vi "Agilent34410A Get Apperture.vi"(8 "error in (no error)":errorcluster, 10 "DMM Function":T2, 11 "VISA Rsrc":refnum<visa-resource-name>="SR530") -> (0 "error out":errorcluster, 1 "Aperture (s)":dbl, 2 "NPLC Val":dbl, 3 "VISA Rsrc Out":refnum<visa-resource-name>="GPIB0::12::INSTR", 4 "ChaineRep":string caption="Chaîne de Réponse", 5 "Apperture Enable":bool caption="App Enable", 6 "NPLC":T1(ring))   [LabVIEW 2019]
uses:
  <userlib>/Agilent34410A/Agilent34410A DMM_Func.ctl
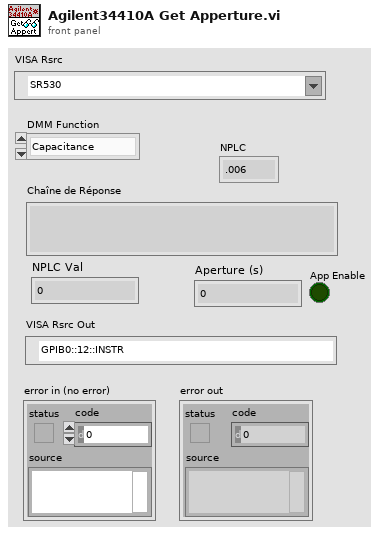
[diagram p1: front panel]
types:
  T1 = enum16{".006", ".02", ".06", ".2", "1", "2", "10", "100"}
  T2 = typedef "Agilent34410A DMM_Func.ctl" = enum16{"Capacitance", "Continuity", "Current AC", "Current", "Diode", "Frequency", "4W Resistance", "Period", "Resistance", "Temperature", "Voltage AC", "Voltage"}
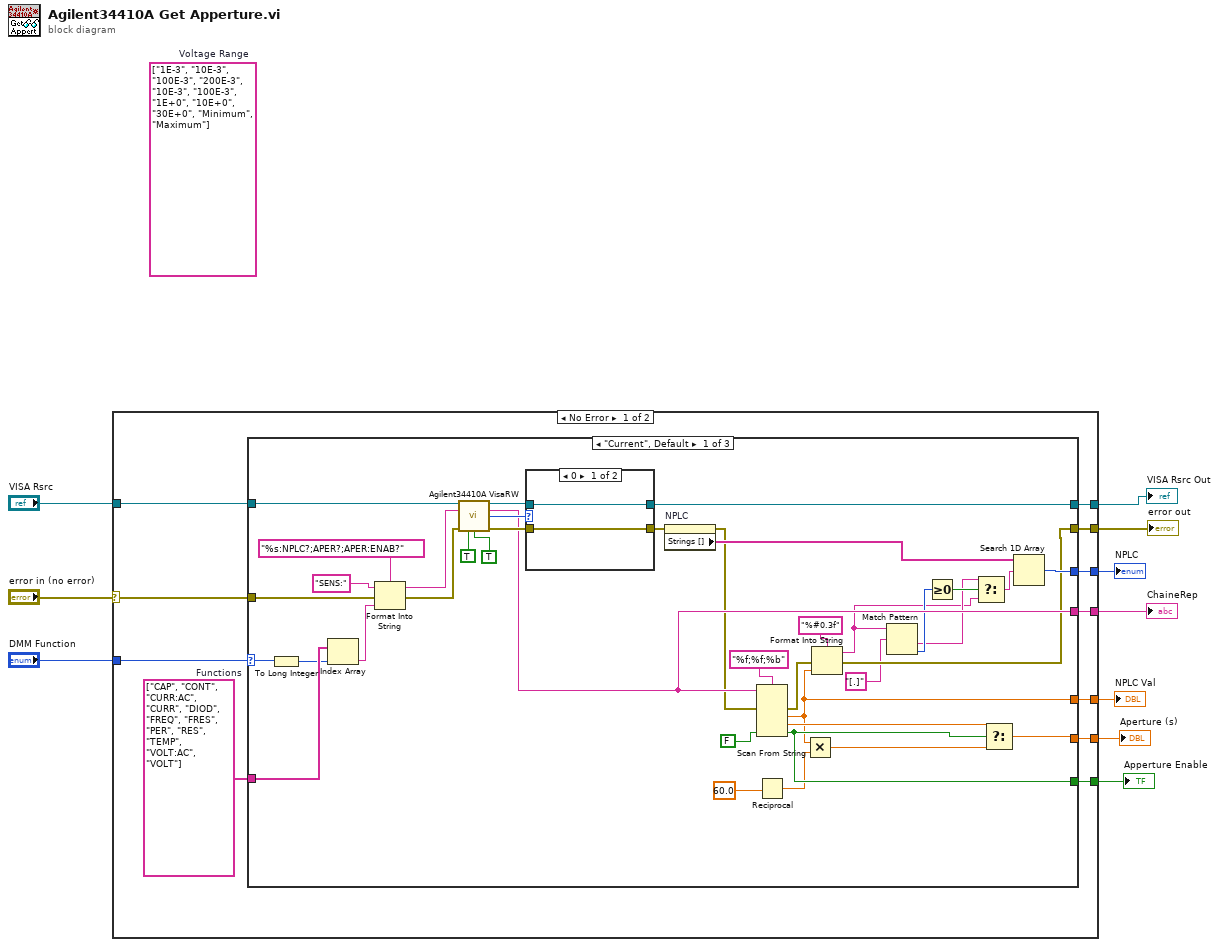
[diagram p0: block diagram]
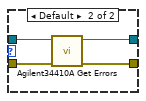
[diagram p2: hidden frame]
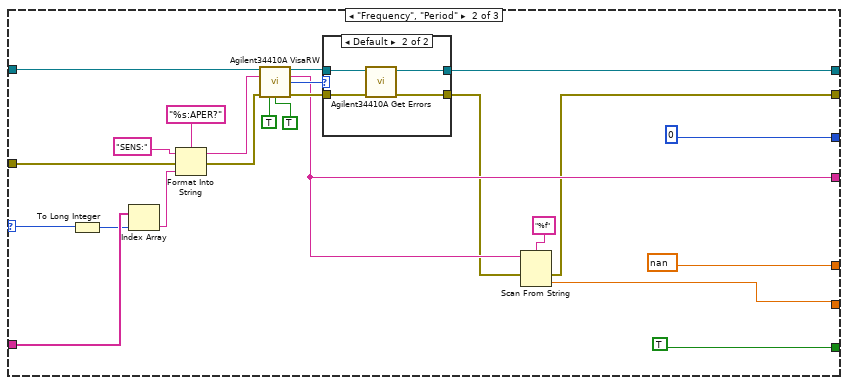
[diagram p3: hidden frame]
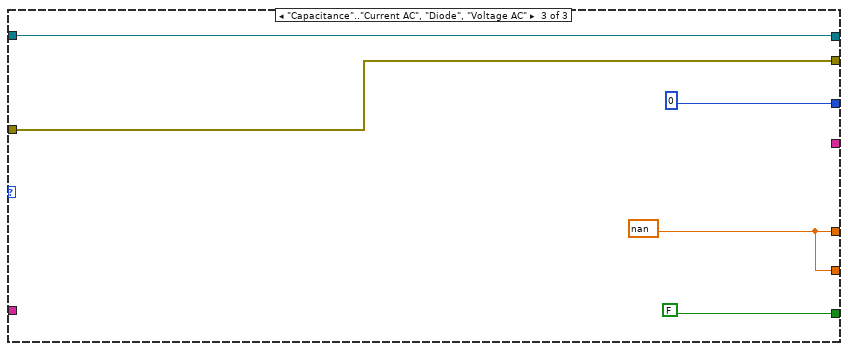
[diagram p5: hidden frame]
diagram:
  (unwired) string[] ["1E-3", "10E-3", "100E-3", "200E-3", "10E-3", "100E-3", "1E+0", "10E+0", "30E+0", "Minimum", "Maximum"]  # Voltage Range
  n1 = case shown="No Error" "error in (no error)" {
    selector: "error in (no error)" -> [w20 w102]
    tunnel: "VISA Rsrc" -> [w21 w103]
    tunnel: [w18 w102] -> w8
    tunnel: [w19 w103] -> w7
    tunnel: [w16 _] -> w6
    tunnel: "DMM Function" -> [w15 _]
    tunnel: [w14 _] -> w4
    tunnel: [w13 _] -> w3
    tunnel: [w12 _] -> w2
    tunnel: [w11 _] -> w1
    frame No Error {
      w17 = string[] ["CAP", "CONT", "CURR:AC", "CURR", "DIOD", "FREQ", "FRES", "PER", "RES", "TEMP", "VOLT:AC", "VOLT"]  # Functions
      n2 = case shown="\"Current\", Default" w15 {
        selector: w15 -> [w47 w77 _]
        tunnel: w21 -> [w60 w90 w101]
        tunnel: w20 -> [w57 w87 w100]
        tunnel: [w51 w81 w101] -> w19
        tunnel: [w28 w71 w100] -> w18
        tunnel: w17 -> [w50 w80 _]
        tunnel: [w33 w75 _] -> w16
        tunnel: [w40 w69 w99] -> w14
        tunnel: [w32 nan w99] -> w13
        tunnel: [w42 TRUE FALSE] -> w12
        tunnel: [w34 0 ("index of element") 0 ("index of element")] -> w11
        frame "Current", Default {
          n3 = To Long Integer(number=w47) -> (32bit integer=w46:i32)
          n4 = Index Array(array=w50, index=w46) -> (element=w49:string)
          n5 = Format Into String(format string="%s:NPLC?;APER?;APER:ENAB?" ("string (\"\")"), initial string="SENS:" ("string (\"\")"), error in=w57, w49) -> (resulting string=w48:string, error out=w56:errorcluster)
          n6 = call <userlib>:"Agilent34410A VisaRW.vi"("VISA Rsrc"=w60, "ChaineCom"=w48, "error in (no error)"=w56, "Lecture?(T)"=TRUE, "Poll?(F)"=TRUE) -> ("VISA Rsrc Out"=w52:refnum<visa-resource-name>, "ChaineRep"=w33:string, "octet d'état"=w53:u16, "error out"=w54:errorcluster)  [unwired: 6 in, 1 out]
          n7 = case shown="0" w53 {
            tunnel: w52 -> [w62 w66]
            tunnel: w54 -> [w61 w65]
            tunnel: [w61 w64] -> w35
            tunnel: [w62 w63] -> w51
            frame 0 {
            }
            frame Default {
              n8 = call <userlib>:"Agilent34410A Get Errors.vi"("error in (no error)"=w65, "VISA Rsrc"=w66) -> ("error out"=w64:errorcluster, "VISA Rsrc Out"=w63:refnum<visa-resource-name>)  [unwired: 7 in, 1 out]
            }
          }
          n9 = property on="NPLC" class="Énum (strict)"(error in=w35) -> (error out=w29:errorcluster, "Strings []"=w36:string[])  [unwired: 1 in, 1 out]
          n10 = Scan From String(format string="%f;%f;%b" ("chaîne de format"), input string=w33, error in=w29, default 3=FALSE) -> (error out=w30:errorcluster, output 1=w32:dbl, output 2=w41:dbl, output 3=w42:bool)  [unwired: 3 in, 2 out]
          n11 = Reciprocal(x=60.0 ("y")) -> (1/x=w38:dbl)
          n12 = Multiply(x=w32, y=w38) -> (x*y=w37:dbl)
          n13 = Format Into String(format string="%#0.3f" ("chaîne de format"), error in=w30, w32) -> (resulting string=w22:string, error out=w28:errorcluster)  [unwired: 1 in]
          n14 = Match Pattern(string=w22, regular expression="[.]" ("expression régulière")) -> (after substring=w24:string, offset past match=w25:i32)  [unwired: 1 in, 2 out]
          n15 = Greater Or Equal To 0?(x=w25) -> (x >= 0?=w27:bool)
          n16 = Select(t=w24, s=w27, f=w22) -> (s? t:f=w26:string)
          n17 = Select(t=w41, s=w42, f=w37) -> (s? t:f=w40:dbl)
          n18 = Search 1D Array(1D array=w36, element=w26) -> (index of element=w34:i32)  [unwired: 1 in]
        }
        frame "Frequency", "Period" {
          n19 = To Long Integer(number=w77) -> (32bit integer=w76:i32)
          n20 = Index Array(array=w80, index=w76) -> (element=w79:string)
          n21 = Format Into String(format string="%s:APER?" ("string (\"\")"), initial string="SENS:" ("string (\"\")"), error in=w87, w79) -> (resulting string=w78:string, error out=w86:errorcluster)
          n22 = call <userlib>:"Agilent34410A VisaRW.vi"("VISA Rsrc"=w90, "ChaineCom"=w78, "error in (no error)"=w86, "Lecture?(T)"=TRUE, "Poll?(F)"=TRUE) -> ("VISA Rsrc Out"=w82:refnum<visa-resource-name>, "ChaineRep"=w75:string, "octet d'état"=w83:u16, "error out"=w84:errorcluster)  [unwired: 6 in, 1 out]
          n23 = case shown="Default" w83 {
            tunnel: w82 -> [w92 w96]
            tunnel: w84 -> [w91 w95]
            tunnel: [w91 w94] -> w72
            tunnel: [w92 w93] -> w81
            frame 0 {
            }
            frame Default {
              n24 = call <userlib>:"Agilent34410A Get Errors.vi"("error in (no error)"=w95, "VISA Rsrc"=w96) -> ("error out"=w94:errorcluster, "VISA Rsrc Out"=w93:refnum<visa-resource-name>)  [unwired: 7 in, 1 out]
            }
          }
          n25 = Scan From String(format string="%f" ("chaîne de format"), input string=w75, error in=w72) -> (error out=w71:errorcluster, output 1=w69:dbl)  [unwired: 2 in, 2 out]
        }
        frame "Capacitance".."Current AC", "Diode", "Voltage AC" {
          w99 = nan
        }
      }
    }
    frame Error {
    }
  }
  "error out" <- w8
  "VISA Rsrc Out" <- w7
  "ChaineRep" <- w6
  "Aperture (s)" <- w4
  "NPLC Val" <- w3
  "Apperture Enable" <- w2
  "NPLC" <- w1
